vi "ReadTemperature.vi"(0 "reference in":refnum<class "SHT21.lvclass">, 5 "error in (no error)":errorcluster, 6 "LINX Resource":T1={"IO"=enum."Remote", "Interface"=enum."Serial", "LINX Device Config"={"Interface"=enum."Serial", "COM Port"="COM13", "TCP Configuration"={"IP Address"="", "Port"=0}, "Device Family"=1, "Device ID"=1, "Device Name"="myRIO-1900", "TCP Ref"=refnum, "Channels"={"DI"=[0, 1, 2, 3, 4, 5, 6, 7, 8, 9, 10, 11, 12, 13, 14, 15, 16, 17, 18, 19, 20, 21, 22, 23, 24, 25, 26, 27, 28, 29, 30, 31, 32, 33, 34, 35, 36, 37, 38, 39, 40, 41, 42, 43, 44, 45, 46], "DO"=[0, 1, 2, 3, 4, 5, 6, 7, 8, 9, 10, 11, 12, 13, 14, 15, 16, 17, 18, 19, 20, 21, 22, 23, 24, 25, 26, 27, 28, 29, 30, 31, 32, 33, 34, 35, 36, 37, 38, 39, 40, 41, 42, 43, 44, 45, 46], "AI"=[0, 1, 2, 3, 4, 5, 6, 7, 8, 9, 10, 11], "AO"=[], "PWM"=[3, 5, 6, 9, 10], "QE"=[], "UART"=[0, 1], "I2C 2"=[0], "SPI"=[0], "CAN"=[], "Servo"=[], "AI Ref (V)"=0.0, "AI Resolution (Bits)"=0, "AO Ref (V)"=0.0, "AO Resolution (Bits)"=0}}}) -> (12 "LINX Resource":T1={"IO"=enum."Remote", "Interface"=enum."Serial", "LINX Device Config"={"Interface"=enum."Serial", "COM Port"="COM13", "TCP Configuration"={"IP Address"="", "Port"=0}, "Device Family"=1, "Device ID"=1, "Device Name"="myRIO-1900", "TCP Ref"=refnum, "Channels"={"DI"=[0, 1, 2, 3, 4, 5, 6, 7, 8, 9, 10, 11, 12, 13, 14, 15, 16, 17, 18, 19, 20, 21, 22, 23, 24, 25, 26, 27, 28, 29, 30, 31, 32, 33, 34, 35, 36, 37, 38, 39, 40, 41, 42, 43, 44, 45, 46], "DO"=[0, 1, 2, 3, 4, 5, 6, 7, 8, 9, 10, 11, 12, 13, 14, 15, 16, 17, 18, 19, 20, 21, 22, 23, 24, 25, 26, 27, 28, 29, 30, 31, 32, 33, 34, 35, 36, 37, 38, 39, 40, 41, 42, 43, 44, 45, 46], "AI"=[0, 1, 2, 3, 4, 5, 6, 7, 8, 9, 10, 11], "AO"=[], "PWM"=[3, 5, 6, 9, 10], "QE"=[], "UART"=[0, 1], "I2C 2"=[0], "SPI"=[0], "CAN"=[], "Servo"=[], "AI Ref (V)"=0.0, "AI Resolution (Bits)"=0, "AO Ref (V)"=0.0, "AO Resolution (Bits)"=0}}}, 14 "reference out":refnum<class "SHT21.lvclass">, 15 "Temperature":dbl, 17 "Data Temp":u8[](array[numeric]), 19 "error out":errorcluster)   [LabVIEW 2019, in "SHT21.lvclass"]
uses:
  SHT21.lvclass
  <vilib>/MakerHub/LINX/Private/Type Defs/LINX Ref.ctl
  <vilib>/MakerHub/LINX/Private/Type Defs/Platform.ctl
  <vilib>/MakerHub/LINX/Private/Type Defs/Interface.ctl
  <vilib>/MakerHub/LINX/Private/Device/Type Defs/LINX Device Config.ctl
  <vilib>/MakerHub/LINX/Private/Device/Type Defs/TCP Config.ctl
  <vilib>/MakerHub/LINX/Private/Device/Type Defs/Channels.ctl
  <vilib>/MakerHub/LINX/Private/Local IO/LinxI2cWrite.vi
  <vilib>/MakerHub/LINX/Public/Utilities/Check Channel.vi
  <vilib>/MakerHub/LINX/Private/Local IO/Handle Errors.vi
  <vilib>/MakerHub/LINX/Private/Utilties/Generate Error.vi
  <vilib>/MakerHub/LINX/LMH-LINX.lvlib
  <vilib>/MakerHub/LINX/Private/Device/Device.lvlib
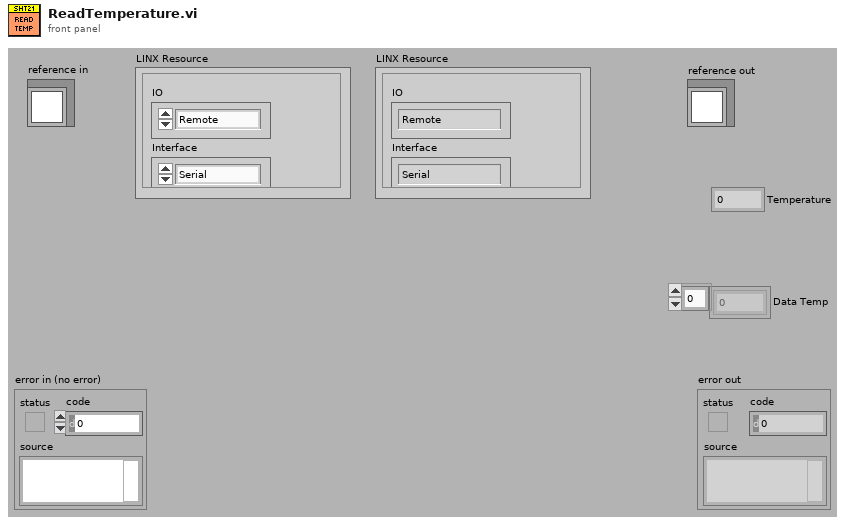
[diagram p1: front panel]
types:
  T1 = typedef "LMH-LINX.lvlib/LINX Ref.ctl" = cluster{"IO":T2, "Interface":T3, "LINX Device Config":T4}
  T2 = typedef "LMH-LINX.lvlib/Platform.ctl" = enum16{"Remote", "Local"}
  T3 = typedef "LMH-LINX.lvlib/Interface.ctl" = enum16{"Serial", "TCP"}
  T4 = typedef "LMH-LINX.lvlib/Device.lvlib/LINX Device Config.ctl" = cluster{"Interface":T3, "COM Port":refnum<visa-resource-name>, "TCP Configuration":T5, "Device Family":u8, "Device ID":u8, "Device Name":string, "TCP Ref":refnum<k5>, "Channels":T6}
  T5 = typedef "LMH-LINX.lvlib/Device.lvlib/TCP Config.ctl" = cluster{"IP Address":string, "Port":u16}
  T6 = typedef "LMH-LINX.lvlib/Channels.ctl" = cluster{"DI":u8[], "DO":u8[], "AI":u8[], "AO":u8[], "PWM":u8[], "QE":u8[], "UART":u8[], "I2C 2":u8[], "SPI":u8[], "CAN":u8[], "Servo":u8[], "AI Ref (V)":dbl, "AI Resolution (Bits)":u8, "AO Ref (V)":dbl, "AO Resolution (Bits)":u8}
  T7 = typedef "SHT21.lvclass/ObjectAttributes.ctl" = cluster{"I2C Slave Address (0)":u8, "I2C Channel (0)":u8, "T Offset":dbl, "RH Offset":dbl}
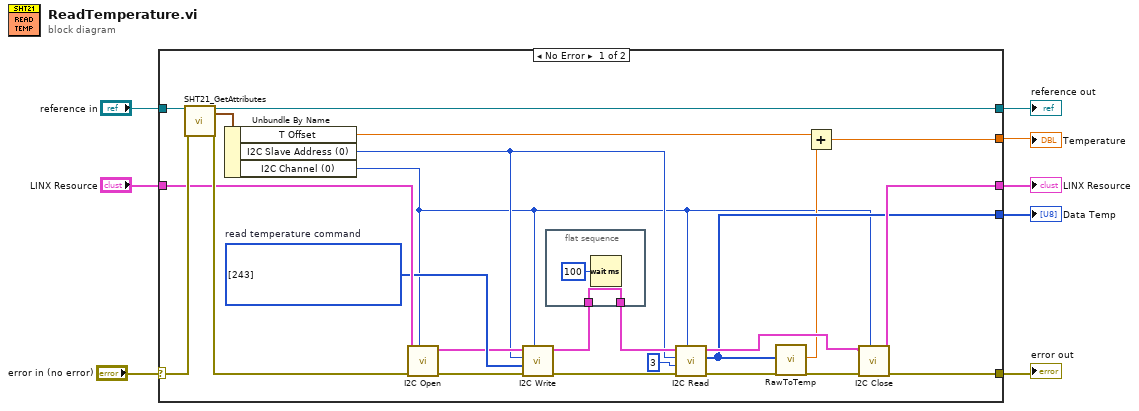
[diagram p0: block diagram]
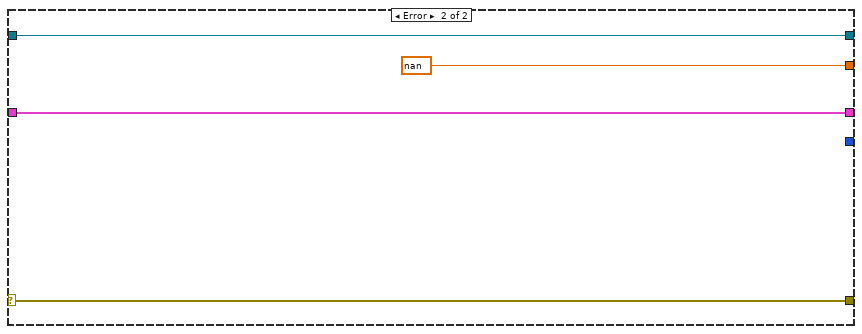
[diagram p2: hidden frame]
diagram:
  n1 = case shown="No Error" "error in (no error)" {
    selector: "error in (no error)" -> [w32 w38]
    tunnel: [w27 w38] -> w7
    tunnel: [w30 w37] -> w5
    tunnel: "reference in" -> [w31 w37]
    tunnel: "LINX Resource" -> [w28 w36]
    tunnel: [w26 w36] -> w3
    tunnel: [w24 nan] -> w2
    tunnel: [w15 _] -> w1
    frame No Error {
      w22 = u8[] [243]  # read temperature command
      n2 = call "SHT21_GetAttributes.vi"("reference in"=w31, "error in (no error)"=w32) -> ("reference out"=w30:refnum<class "SHT21.lvclass">, "Data"=w25:T7, "error out"=w29:errorcluster)  [unwired: 14 in, 1 out]
      n3 = Unbundle By Name(w25) -> ("T Offset"=w23:dbl, "I2C Slave Address (0)"=w10:u8, "I2C Channel (0)"=w9:u8)
      n4 = call <vilib>:"I2C Open.vi"("I2C Channel (0)"=w9, "Error In"=w29, "LINX Resource"=w28) -> ("Error Out"=w11:errorcluster, "LINX Resource"=w21:T1)  [unwired: 7 in]
      n5 = call <vilib>:"I2C Write.vi"("I2C Channel"=w9, "Error In"=w11, "Data"=w22, "I2C Slave Address (0)"=w10, "LINX Resource"=w21) -> ("Error Out"=w18:errorcluster, "LINX Resource"=w13:T1)  [unwired: 5 in]
      n6 = flat-sequence {
        tunnel: [w34] -> w12
        tunnel: w13 -> [w34]
        frame #0 {
          n7 = Wait (ms)(milliseconds to wait=u32 100) -> ()  [unwired: 1 out]
        }
      }
      n8 = call <vilib>:"I2C Read.vi"("I2C Channel"=w9, "Error In"=w18, "Bytes To Read"=u8 3, "I2C Slave Address (0)"=w10, "LINX Resource"=w12) -> ("Error Out"=w19:errorcluster, "Data"=w15:u8[], "LINX Resource"=w16:T1)  [unwired: 4 in]
      n9 = call "RawToTemp.vi"("Data"=w15, "error in (no error)"=w19) -> ("Temperature"=w14:dbl, "error out"=w17:errorcluster)  [unwired: 16 in]
      n10 = Add(x=w23, y=w14) -> (x+y=w24:dbl)
      n11 = call <vilib>:"I2C Close.vi"("I2C Channel (0)"=w9, "Error In"=w17, "LINX Resource"=w16) -> ("Error Out"=w27:errorcluster, "LINX Resource"=w26:T1)  [unwired: 7 in]
    }
    frame Error {
    }
  }
  "error out" <- w7
  "reference out" <- w5
  "LINX Resource" <- w3
  "Temperature" <- w2
  "Data Temp" <- w1
